vi "AVI to TIFF.vi"() -> ()   [LabVIEW 2012]
panel:
  in  "Delete AVI?":bool
  out "error out":errorcluster
  in  "Error in (no error)":errorcluster
  in  "AVI Path":path
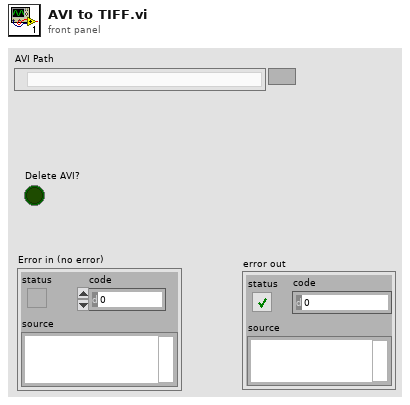
[diagram p1: front panel]
types:
  T1 = typedef "IMAQ Image.ctl" = refnum<image>
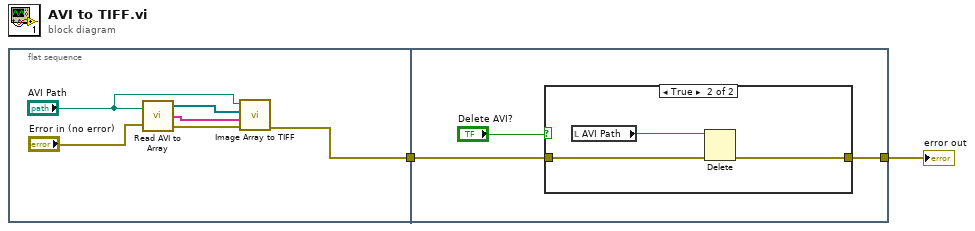
[diagram p0: block diagram]
diagram:
  n1 = flat-sequence {
    tunnel: [w3] -> w2
    tunnel: w2 -> [w10]
    tunnel: [w9] -> w1
    frame #0 {
      n2 = call "Read AVI to Array.vi"("AVI Path"="AVI Path", "Error in (no error)"="Error in (no error)") -> ("Image Array"=w8:T1[], "Data Array"=w7:string[], "Error out"=w6:errorcluster)
      n3 = call "Image Array to TIFF.vi"("error in"=w6, "Data Array"=w7, "Image Array"=w8, "Destination Image File"="AVI Path") -> ("error out"=w3:errorcluster)  [unwired: 7 in]
    }
    frame #1 {
      n4 = case shown="True" "Delete AVI?" {
        tunnel: w10 -> [w12 w14]
        tunnel: [w12 w13] -> w9
        frame False {
        }
        frame True {
          n5 = local read "AVI Path"() -> (w15:path)
          n6 = Delete(path (use dialog)=w15, error in=w14) -> (error out=w13:errorcluster)  [unwired: 3 in, 2 out]
        }
      }
    }
  }
  "error out" <- w1
